vi "Init.vi"(8 "error in (no error)":errorcluster, 10 "Channel":i16, 11 "TrialBasedExperiment in":refnum<class "TrialBasedExperiment.lvclass">) -> (0 "error out":errorcluster, 3 "TrialBasedExperiment out":refnum<class "TrialBasedExperiment.lvclass">)   [LabVIEW 2011, in "TrialBasedExperiment.lvclass"]
uses:
  TrialBasedExperiment.lvclass
  Acquisition/AcquistionObject/AcquistionObject.lvclass
panel:
  in  "Subject":string(combo)="Ben"
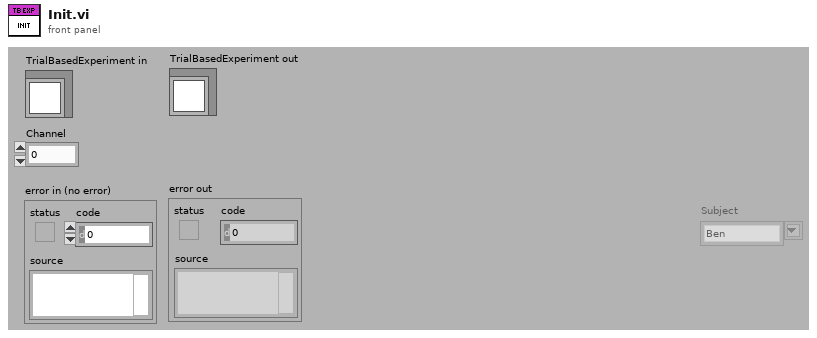
[diagram p1: front panel]
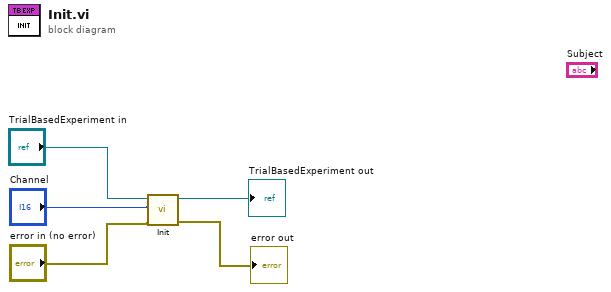
[diagram p0: block diagram]
diagram:
  n1 = call-parent "Init.vi"("error in (no error)"="error in (no error)", "Channel"="Channel", "AcquistionObject in"="TrialBasedExperiment in") -> ("error out"=→"error out":errorcluster, "AcquistionObject out"=→"TrialBasedExperiment out":refnum<class "TrialBasedExperiment.lvclass">)  [unwired: 7 in]
